vi "WaitPass3.vi"(7 "AI Parameters":T1={"GotoKick"={"Dist do cone a frente"=150.0, "attacker farback"=1500.0, "Perto"=300.0, "min dist to kick"=150.0, "kick eps"=0.0, "Time to transition"=0.05}, "Attacker"={"CC chute"=0.09, "CC passe"=0.045, "Kick Force"=100.0, "ball-robot Kick"=200.0, "ball-robot Pass"=0.3, "drible\nAttk"=FALSE}, "Defender"={"D max"=1700.0, "Vel p/ robô av"=1000.0, "Kick Force"=100.0, "D atk-def"=0.0, "D farback"=0.0, "drible\ndef"=FALSE, "drible\ngoalie"=FALSE}, "Timeout"={"Field/v in x"=6.0, "Dist Robots"=300, "Dist up in y"=300}, "Pose Striker"={"dist"=200.0, "Numeric"=-4.0, "dist 2"=200.0, "drible\nstriker"=FALSE}, "Dist Stop"=300.0, "D ball out"=200, "D central gap "=150.0, "T pass"=0.0, "Force ++"=0.0, "range kick"=0.0, "Chute alto"=TRUE, "Marcador novo"=TRUE, "drible"=FALSE, "D drible"=300.0} {"D drible" format="%#_13g"; "D central gap" format="%#_13g"; "Dist Stop" format="%#_13g"; "Pose Striker"."Numeric" format="%#_13g"; "Defender"."Kick Force" format="%#_13g"; "Defender"."Vel p/ robô av" format="%#_13g"; "Attacker"."ball-robot Kick" format="%#_13g"; "Attacker"."Kick Force" format="%#_13g"; "Attacker"."CC passe" format="%#_13g"; "Attacker"."CC chute" format="%#_13g"; "GotoKick"."kick eps" format="%#_13g"; "GotoKick"."min dist to kick" format="%#_13g"; "GotoKick"."Perto" format="%#_13g"; "GotoKick"."attacker farback" format="%#_13g"; "GotoKick"."Dist do cone a frente" format="%#_13g"}, 8 "Best Y Inverso":dbl[](array[numeric]), 9 "Target":dbl[](array[numeric]), 10 "balls":T7[](array[typedef])=[{"x"=-2165.869384765625, "y"=510.4085693359375, "timestamp"=timestamp(2082758857.4639893 s since 1904-01-01), "Vel_x"=0.0, "Vel_y"=0.0, "Pos Bola Est"=[]}], 11 "Robot in":T2) -> (2 "Robot out":T2)   [LabVIEW 2017]
uses:
  Core/AI Robot.ctl
  Functions Enum.ctl
  AttackerStates.ctl
  Path Planning/RRT/PathDests.ctl
  Path Planning/RRT/PathDest.ctl
  Core/AI Ball.ctl
  AI Parameters.ctl
  <vilib>/Analysis/_algsub.llb/Real Vector Norm.vi
  <vilib>/Analysis/NI_AALPro.lvlib
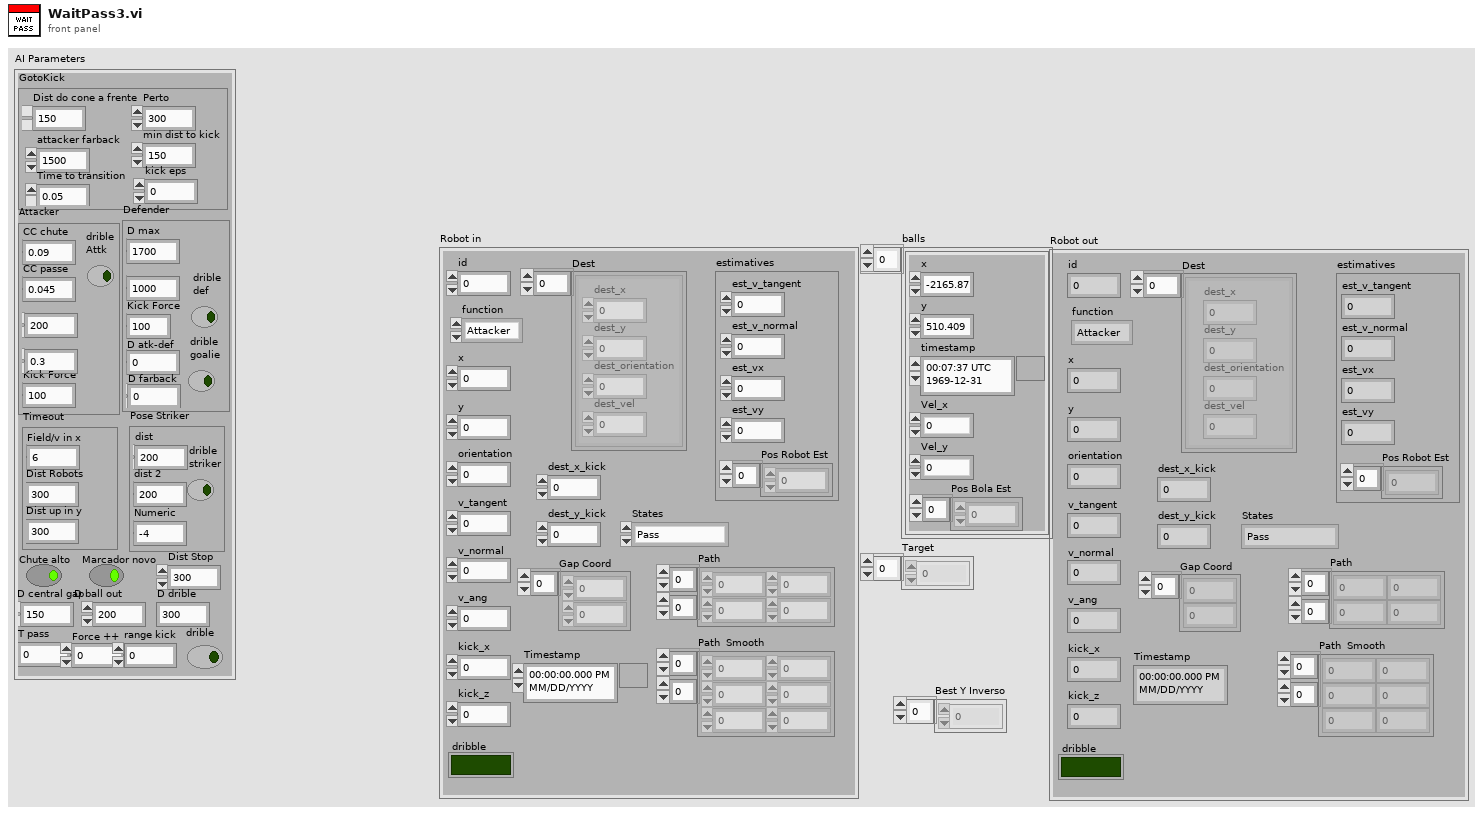
[diagram p1: front panel]
types:
  T1 = typedef "AI Parameters.ctl" = cluster{"GotoKick":cluster{"Dist do cone a frente":dbl, "attacker farback":dbl, "Perto":dbl, "min dist to kick":dbl, "kick eps":dbl, "Time to transition":dbl}, "Attacker":cluster{"CC chute":dbl, "CC passe":dbl, "Kick Force":dbl, "ball-robot Kick":dbl, "ball-robot Pass":dbl, "drible\nAttk":bool}, "Defender":cluster{"D max":dbl, "Vel p/ robô av":dbl, "Kick Force":dbl, "D atk-def":dbl, "D farback":dbl, "drible\ndef":bool, "drible\ngoalie":bool}, "Timeout":cluster{"Field/v in x":dbl, "Dist Robots":u32, "Dist up in y":u32}, "Pose Striker":cluster{"dist":dbl, "Numeric":dbl, "dist 2":dbl, "drible\nstriker":bool}, "Dist Stop":dbl, "D ball out":i32, "D central gap ":dbl, "T pass":dbl, "Force ++":dbl, "range kick":dbl, "Chute alto":bool, "Marcador novo":bool, "drible":bool, "D drible":dbl}
  T2 = typedef "AI Robot.ctl" = cluster{"id":u32, "function":T3, "x":dbl, "y":dbl, "orientation":dbl, "v_tangent":dbl, "v_normal":dbl, "v_ang":dbl, "kick_x":dbl, "kick_z":dbl, "dribble":bool, "Timestamp":timestamp, "estimatives":cluster{"est_v_tangent":dbl, "est_v_normal":dbl, "est_vx":dbl, "est_vy":dbl, "Pos Robot Est":dbl[]}, "dest_x_kick":dbl, "dest_y_kick":dbl, "Gap Coord":dbl[], "States":T4, "Path ":dbl[][], "Path  Smooth":dbl[][], "Dest":T5}
  T3 = typedef "Functions Enum.ctl" = enum16{"Attacker", "Goalie", "Defender", "Striker", "Goto 0", "Dummy", "Kicker", "ZigZag 0", "ZigZag 1", "ZigZag 2", "ZigZag 3", "ZigZag 4", "ZigZag 5", "ZigZag 6", "ZigZag 7", "ZigZag 8", ""}
  T4 = typedef "AttackerStates.ctl" = enum16{"Pass", "GoToTangent", "BallGetting", "GoToKick", ""}
  T5 = typedef "PathDests.ctl" = T6[]
  T6 = typedef "PathDest.ctl" = cluster{"dest_x":dbl, "dest_y":dbl, "dest_orientation":dbl, "dest_vel":dbl}
  T7 = typedef "AI Ball.ctl" = cluster{"x":dbl, "y":dbl, "timestamp":timestamp, "Vel_x":dbl, "Vel_y":dbl, "Pos Bola Est":dbl[]}
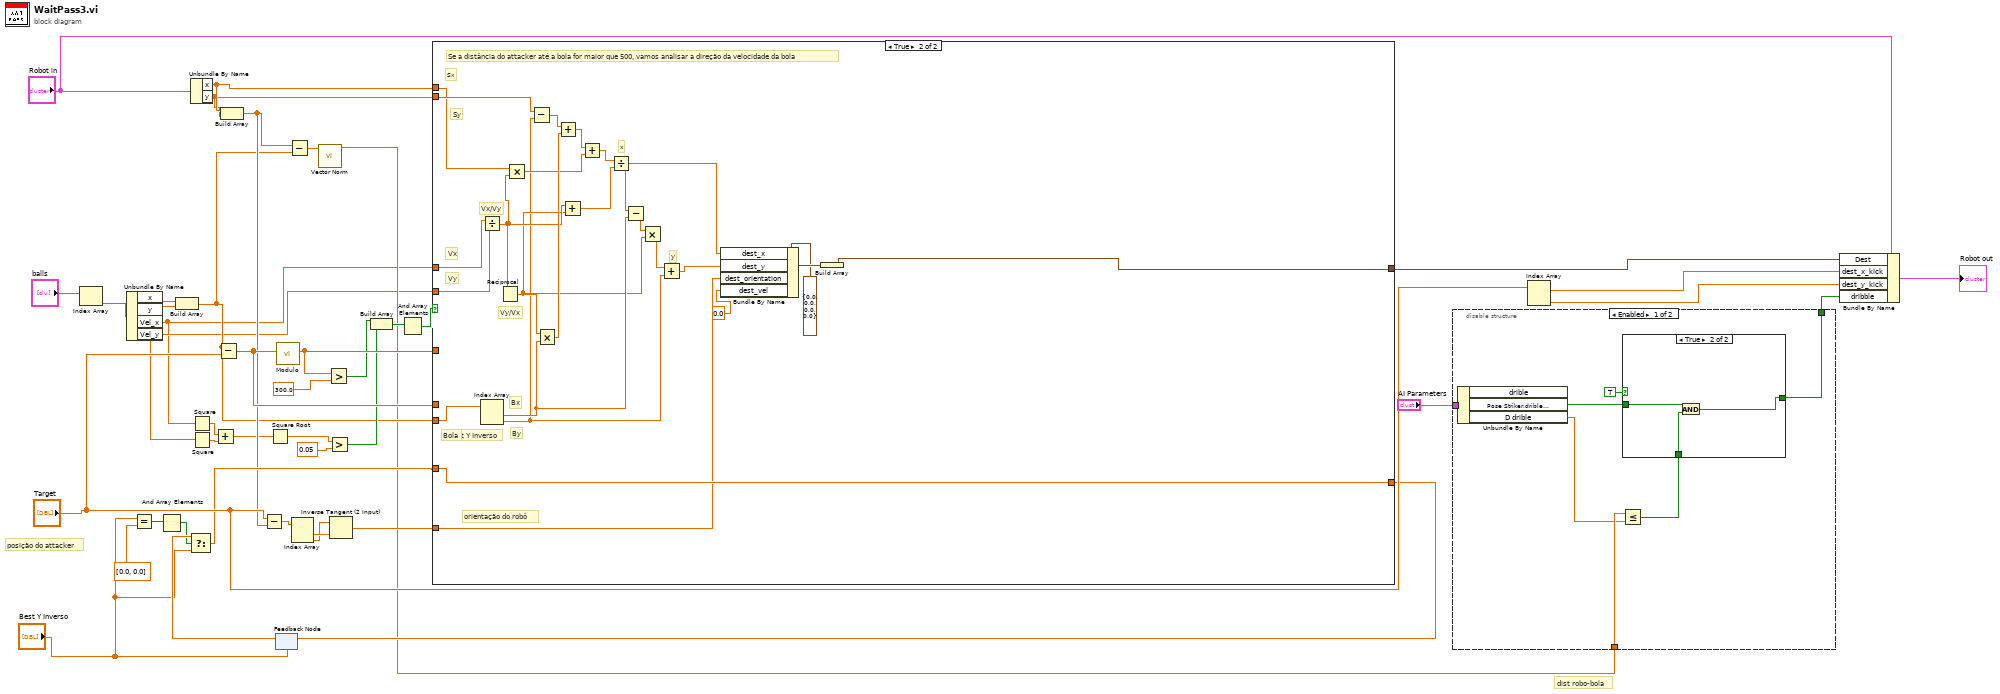
[diagram p0: block diagram]
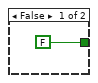
[diagram p2: hidden frame]
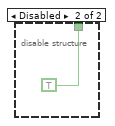
[diagram p3: hidden frame]
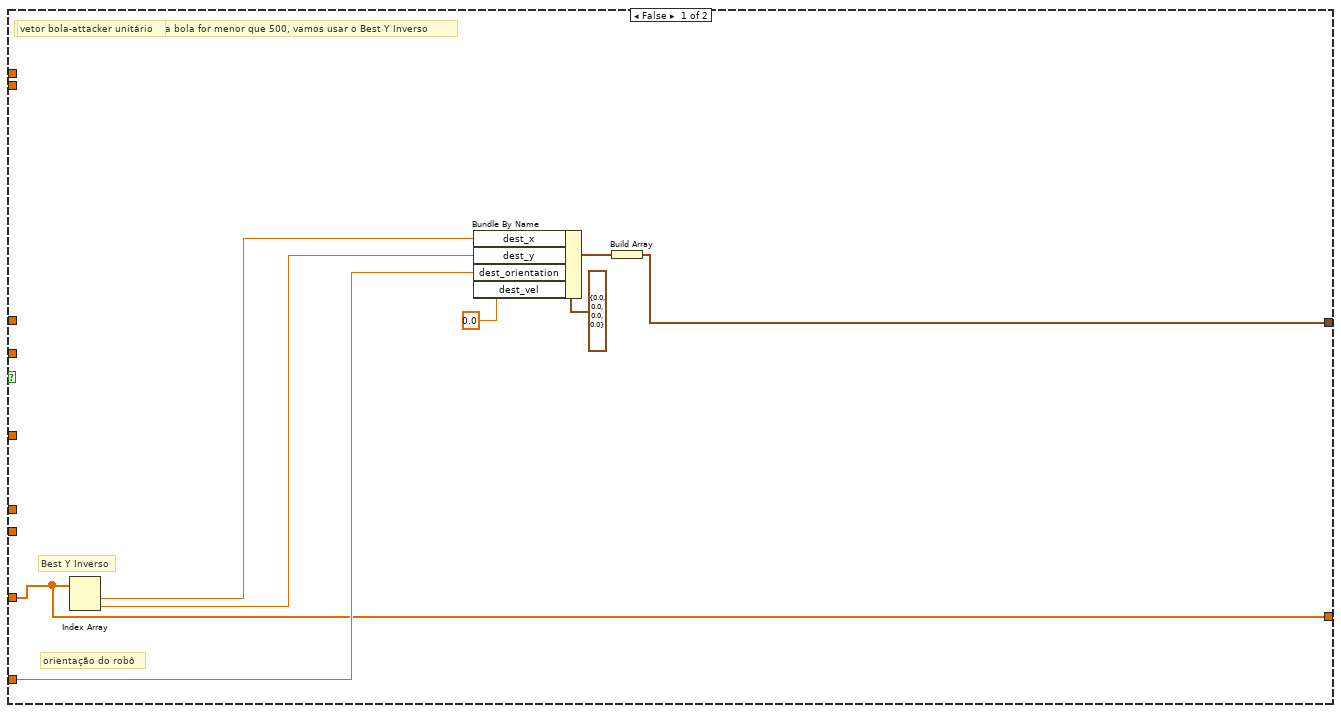
[diagram p4: hidden frame]
diagram:
  # "dist robo-bola"
  # "posição do attacker"
  n1 = Index Array(array="balls") -> (element=w42:T7)  [unwired: 1 in]
  n2 = Unbundle By Name(w42) -> ("x"=w41:dbl, "y"=w40:dbl, "Vel_x"=w5:dbl, "Vel_y"=w6:dbl)
  n3 = Equal?(x="Best Y Inverso", y=dbl[] [0.0, 0.0] ("FinalPosition")) -> (x = y?=w16:bool[])
  n4 = And Array Elements(Boolean array=w16) -> (logical AND=w15:bool)
  n5 = Build Array(w41, w40) -> (w12:dbl[])
  n6 = Unbundle By Name("Robot in") -> ("x"=w34:dbl, "y"=w33:dbl)
  n7 = Square(x=w5) -> (x^2=w3:dbl)
  n8 = Square(x=w6) -> (x^2=w2:dbl)
  n9 = Add(x=w3, y=w2) -> (x+y=w1:dbl)
  n10 = Subtract(x=w12, y="Target") -> (x-y=w27:dbl[])
  n11 = Build Array(w34, w33) -> (w13:dbl[])
  n12 = Subtract(x="Target", y=w13) -> (x-y=w35:dbl[])
  n13 = Square Root(x=w1) -> (sqrt(x)=w4:dbl)
  n14 = feedback #1("Best Y Inverso") -> (w19:dbl[])
  n15 = Select(t=w19, s=w15, f="Best Y Inverso") -> (s? t:f=w18:dbl[])
  n16 = call "Modulo.vi"("2D vector"=w27) -> ("Modulo"=w38:dbl)  [unwired: 10 in]
  n17 = Subtract(x=w13, y=w12) -> (x-y=w11:dbl[])
  n18 = Index Array(array=w35) -> (element #1=w37:dbl, element #2=w36:dbl)  [unwired: 2 in]
  n19 = call-poly <vilib>:"Vector Norm.vi"("Input Vector"=w11) -> ("norm"=w8:dbl)  [unwired: 9 in, 1 out]
  n20 = Greater?(x=w38, y=300.0) -> (0:w26:bool)
  n21 = Greater?(x=w4, y=0.05 ("x")) -> (0:w25:bool)
  n22 = Inverse Tangent (2 Input)(1:w37, 2:w36) -> (0:w32:dbl)
  n23 = Build Array(w26, w25) -> (w24:bool[])
  n24 = And Array Elements(Boolean array=w24) -> (logical AND=w23:bool)
  n25 = case shown="True" w23 {
    tunnel: w34 -> [_ w64]
    tunnel: w33 -> [_ w67]
    tunnel: w27 -> [_ _]
    tunnel: w38 -> [_ _]
    tunnel: w32 -> [w48 w70]
    tunnel: [w47 w72] -> w30
    tunnel: w5 -> [_ w69]
    tunnel: w6 -> [_ w68]
    tunnel: w12 -> [_ w76]
    tunnel: w18 -> [w44 w71]
    tunnel: [w44 w71] -> w21
    frame False {
      # "Best Y Inverso"
      # "Se a distância do attacker até a bola for menor que 500, vamos usar o Best Y Inverso"
      # "orientação do robô"
      # "vetor bola-attacker unitário"
      n26 = Index Array(array=w44) -> (element #1=w46:dbl, element #2=w45:dbl)  [unwired: 2 in]
      n27 = Bundle By Name(cluster=T6 {"dest_x"=0.0, "dest_y"=0.0, "dest_orientation"=0.0, "dest_vel"=0.0} ("Dest"), "dest_x"=w46, "dest_y"=w45, "dest_orientation"=w48, "dest_vel"=0.0) -> (w50:T6)
      n28 = Build Array(w50) -> (w47:T6[])
    }
    frame True {
      # "y"
      # "x"
      # "Vy/Vx"
      # "Vx/Vy"
      # "By"
      # "Bx"
      # "Best Y Inverso"
      # "Bola"
      # "Vy"
      # "Vx"
      # "orientação do robô"
      # "Sy"
      # "Sx"
      # "Se a distância do attacker até a bola for maior que 500, vamos analisar a direção da velocidade da bola"
      n29 = Divide(x=w69, y=w68) -> (x/y=w61:dbl)
      n30 = Index Array(array=w76) -> (element #1=w58:dbl, element #2=w54:dbl)  [unwired: 2 in]
      n31 = Reciprocal(x=w61) -> (1/x=w56:dbl)
      n32 = Multiply(x=w64, y=w61) -> (x*y=w62:dbl)
      n33 = Subtract(x=w67, y=w54) -> (x-y=w66:dbl)
      n34 = Multiply(x=w56, y=w58) -> (x*y=w65:dbl)
      n35 = Add(x=w66, y=w65) -> (x+y=w63:dbl)
      n36 = Add(x=w61, y=w56) -> (x+y=w59:dbl)
      n37 = Add(x=w63, y=w62) -> (x+y=w60:dbl)
      n38 = Divide(x=w60, y=w59) -> (x/y=w52:dbl)
      n39 = Subtract(x=w52, y=w58) -> (x-y=w57:dbl)
      n40 = Multiply(x=w57, y=w56) -> (x*y=w55:dbl)
      n41 = Add(x=w55, y=w54) -> (x+y=w53:dbl)
      n42 = Bundle By Name(cluster=T6 {"dest_x"=0.0, "dest_y"=0.0, "dest_orientation"=0.0, "dest_vel"=0.0} ("Dest"), "dest_x"=w52, "dest_y"=w53, "dest_orientation"=w70, "dest_vel"=0.0) -> (w75:T6)
      n43 = Build Array(w75) -> (w72:T6[])
    }
  }
  n44 = feedback-in #1(w21) -> ()
  n45 = disable-structure shown="Enabled" {
    disable-tunnel: "AI Parameters" -> [w83 _]
    disable-tunnel: [w82 TRUE] -> w10
    disable-tunnel: w8 -> [w80 _]
    frame Enabled {
      n46 = Unbundle By Name(w83) -> ("Pose Striker.drible\nstriker"=w81:bool, "D drible"=w78:dbl)  [unwired: 1 out]
      n47 = Less Or Equal?(x=w80, y=w78) -> (x <= y?=w79:bool)
      n48 = case shown="True" TRUE {
        tunnel: [FALSE w85] -> w82
        tunnel: w81 -> [_ w87]
        tunnel: w79 -> [_ w86]
        frame False {
        }
        frame True {
          n49 = And(x=w87, y=w86) -> (x .and. y?=w85:bool)
        }
      }
    }
    frame Disabled {
    }
  }
  n50 = Index Array(array="Target") -> (element #1=w29:dbl, element #2=w9:dbl)  [unwired: 2 in]
  n51 = Bundle By Name(cluster="Robot in", "Dest"=w30, "dest_x_kick"=w29, "dest_y_kick"=w9, "dribble"=w10) -> (→"Robot out":T2)
